vi "Rabi.vi"(6 "Gain":dbl=0.65, 7 "resolution (ns)":dbl=0.5, 9 "margin (ns)":i32=10, 11 "Pi pulse duration":dbl[unit]=5.000000000000001e-07) -> (2 "Array size":dbl=1280.0, 3 "Array":dbl[](array[numeric])=[0.0, 0.0, 0.0, 0.0, 0.0, 0.0, 0.0, 0.0, 0.0, 0.0, 0.0, 0.0, 0.0, 0.0, 0.0, 0.0, 0.0, 0.0, 0.0, 0.0, 0.325, 0.325, 0.325, 0.325, 0.325, 0.325, 0.325, 0.325, 0.325, 0.325, 0.325, 0.325, 0.325, 0.325, 0.325, 0.325, 0.325, 0.325, 0.325, 0.325, 0.325, 0.325, 0.325, 0.325, 0.325, 0.325, 0.325, 0.325, 0.325, 0.325, 0.325, 0.325, 0.325, 0.325, 0.325, 0.325, 0.325, 0.325, 0.325, 0.325, 0.325, 0.325, 0.325, 0.325, 0.325, 0.325, 0.325, 0.325, 0.325, 0.325, 0.325, 0.325, 0.325, 0.325, 0.325, 0.325, 0.325, 0.325, 0.325, 0.325, 0.325, 0.325, 0.325, 0.325, 0.325, 0.325, 0.325, 0.325, 0.325, 0.325, 0.325, 0.325, 0.325, 0.325, 0.325, 0.325, 0.325, 0.325, 0.325, 0.325, 0.325, 0.325, 0.325, 0.325, 0.325, 0.325, 0.325, 0.325, 0.325, 0.325, 0.325, 0.325, 0.325, 0.325, 0.325, 0.325, 0.325, 0.325, 0.325, 0.325, 0.325, 0.325, 0.325, 0.325, 0.325, 0.325, 0.325, 0.325, 0.325, 0.325, 0.325, 0.325, 0.325, 0.325, 0.325, 0.325, 0.325, 0.325, 0.325, 0.325, 0.325, 0.325, 0.325, 0.325, 0.325, 0.325, 0.325, 0.325, 0.325, 0.325, 0.325, 0.325, 0.325, 0.325, 0.325, 0.325, 0.325, 0.325, 0.325, 0.325, 0.325, 0.325, 0.325, 0.325, 0.325, 0.325, 0.325, 0.325, 0.325, 0.325, 0.325, 0.325, 0.325, 0.325, 0.325, 0.325, 0.325, 0.325, 0.325, 0.325, 0.325, 0.325, 0.325, 0.325, 0.325, 0.325, 0.325, 0.325, 0.325, 0.325, 0.325, 0.325, 0.325, 0.325, 0.325, 0.325, 0.325, 0.325, 0.325, 0.325, 0.325, 0.325, 0.325, 0.325, 0.325, 0.325, 0.325, 0.325, 0.325, 0.325, 0.325, 0.325, 0.325, 0.325, 0.325, 0.325, 0.325, 0.325, 0.325, 0.325, 0.325, 0.325, 0.325, 0.325, 0.325, 0.325, 0.325, 0.325, 0.325, 0.325, 0.325, 0.325, 0.325, 0.325, 0.325, 0.325, 0.325, 0.325, 0.325, 0.325, 0.325, 0.325, 0.325, 0.325, 0.325, 0.325, 0.325, 0.325, 0.325, 0.325, 0.325, 0.325, 0.325, 0.325, 0.325, 0.325, 0.325, 0.325, 0.325, 0.325, 0.325, 0.325, 0.325, 0.325, 0.325, 0.325, 0.325, 0.325, 0.325, 0.325, 0.325, 0.325, 0.325, 0.325, 0.325, 0.325, 0.325, 0.325, 0.325, 0.325, 0.325, 0.325, 0.325, 0.325, 0.325, 0.325, 0.325, 0.325, 0.325, 0.325, 0.325, 0.325, 0.325, 0.325, 0.325, 0.325, 0.325, 0.325, 0.325, 0.325, 0.325, 0.325, 0.325, 0.325, 0.325, 0.325, 0.325, 0.325, 0.325, 0.325, 0.325, 0.325, 0.325, 0.325, 0.325, 0.325, 0.325, 0.325, 0.325, 0.325, 0.325, 0.325, 0.325, 0.325, 0.325, 0.325, 0.325, 0.325, 0.325, 0.325, 0.325, 0.325, 0.325, 0.325, 0.325, 0.325, 0.325, 0.325, 0.325, 0.325, 0.325, 0.325, 0.325, 0.325, 0.325, 0.325, 0.325, 0.325, 0.325, 0.325, 0.325, 0.325, 0.325, 0.325, 0.325, 0.325, 0.325, 0.325, 0.325, 0.325, 0.325, 0.325, 0.325, 0.325, 0.325, 0.325, 0.325, 0.325, 0.325, 0.325, 0.325, 0.325, 0.325, 0.325, 0.325, 0.325, 0.325, 0.325, 0.325, 0.325, 0.325, 0.325, 0.325, 0.325, 0.325, 0.325, 0.325, 0.325, 0.325, 0.325, 0.325, 0.325, 0.325, 0.325, 0.325, 0.325, 0.325, 0.325, 0.325, 0.325, 0.325, 0.325, 0.325, 0.325, 0.325, 0.325, 0.325, 0.325, 0.325, 0.325, 0.325, 0.325, 0.325, 0.325, 0.325, 0.325, 0.325, 0.325, 0.325, 0.325, 0.325, 0.325, 0.325, 0.325, 0.325, 0.325, 0.325, 0.325, 0.325, 0.325, 0.325, 0.325, 0.325, 0.325, 0.325, 0.325, 0.325, 0.325, 0.325, 0.325, 0.325, 0.325, 0.325, 0.325, 0.325, 0.325, 0.325, 0.325, 0.325, 0.325, 0.325, 0.325, 0.325, 0.325, 0.325, 0.325, 0.325, 0.325, 0.325, 0.325, 0.325, 0.325, 0.325, 0.325, 0.325, 0.325, 0.325, 0.325, 0.325, 0.325, 0.325, 0.325, 0.325, 0.325, 0.325, 0.325, 0.325, 0.325, 0.325, 0.325, 0.325, 0.325, 0.325, 0.325, 0.325, 0.325, 0.325, 0.325, 0.325, 0.325, 0.325, 0.325, 0.325, 0.325, 0.325, 0.325, 0.325, 0.325, 0.325, 0.325, 0.325, 0.325, 0.325, 0.325, 0.325, 0.325, 0.325, 0.325, 0.325, 0.325, 0.325, 0.325, 0.325, 0.325, 0.325, 0.325, 0.325, 0.325, 0.325, 0.325, 0.325, 0.325, 0.325, 0.325, 0.325, 0.325, 0.325, 0.325, 0.325, 0.325, 0.325, 0.325, 0.325, 0.325, 0.325, 0.325, 0.325, 0.325, 0.325, 0.325, 0.325, 0.325, 0.325, 0.325, 0.325, 0.325, 0.325, 0.325, 0.325, 0.325, 0.325, 0.325, 0.325, 0.325, 0.325, 0.325, 0.325, 0.325, 0.325, 0.325, 0.325, 0.325, 0.325, 0.325, 0.325, 0.325, 0.325, 0.325, 0.325, 0.325, 0.325, 0.325, 0.325, 0.325, 0.325, 0.325, 0.325, 0.325, 0.325, 0.325, 0.325, 0.325, 0.325, 0.325, 0.325, 0.325, 0.325, 0.325, 0.325, 0.325, 0.325, 0.325, 0.325, 0.325, 0.325, 0.325, 0.325, 0.325, 0.325, 0.325, 0.325, 0.325, 0.325, 0.325, 0.325, 0.325, 0.325, 0.325, 0.325, 0.325, 0.325, 0.325, 0.325, 0.325, 0.325, 0.325, 0.325, 0.325, 0.325, 0.325, 0.325, 0.325, 0.325, 0.325, 0.325, 0.325, 0.325, 0.325, 0.325, 0.325, 0.325, 0.325, 0.325, 0.325, 0.325, 0.325, 0.325, 0.325, 0.325, 0.325, 0.325, 0.325, 0.325, 0.325, 0.325, 0.325, 0.325, 0.325, 0.325, 0.325, 0.325, 0.325, 0.325, 0.325, 0.325, 0.325, 0.325, 0.325, 0.325, 0.325, 0.325, 0.325, 0.325, 0.325, 0.325, 0.325, 0.325, 0.325, 0.325, 0.325, 0.325, 0.325, 0.325, 0.325, 0.325, 0.325, 0.325, 0.325, 0.325, 0.325, 0.325, 0.325, 0.325, 0.325, 0.325, 0.325, 0.325, 0.325, 0.325, 0.325, 0.325, 0.325, 0.325, 0.325, 0.325, 0.325, 0.325, 0.325, 0.325, 0.325, 0.325, 0.325, 0.325, 0.325, 0.325, 0.325, 0.325, 0.325, 0.325, 0.325, 0.325, 0.325, 0.325, 0.325, 0.325, 0.325, 0.325, 0.325, 0.325, 0.325, 0.325, 0.325, 0.325, 0.325, 0.325, 0.325, 0.325, 0.325, 0.325, 0.325, 0.325, 0.325, 0.325, 0.325, 0.325, 0.325, 0.325, 0.325, 0.325, 0.325, 0.325, 0.325, 0.325, 0.325, 0.325, 0.325, 0.325, 0.325, 0.325, 0.325, 0.325, 0.325, 0.325, 0.325, 0.325, 0.325, 0.325, 0.325, 0.325, 0.325, 0.325, 0.325, 0.325, 0.325, 0.325, 0.325, 0.325, 0.325, 0.325, 0.325, 0.325, 0.325, 0.325, 0.325, 0.325, 0.325, 0.325, 0.325, 0.325, 0.325, 0.325, 0.325, 0.325, 0.325, 0.325, 0.325, 0.325, 0.325, 0.325, 0.325, 0.325, 0.325, 0.325, 0.325, 0.325, 0.325, 0.325, 0.325, 0.325, 0.325, 0.325, 0.325, 0.325, 0.325, 0.325, 0.325, 0.325, 0.325, 0.325, 0.325, 0.325, 0.325, 0.325, 0.325, 0.325, 0.325, 0.325, 0.325, 0.325, 0.325, 0.325, 0.325, 0.325, 0.325, 0.325, 0.325, 0.325, 0.325, 0.325, 0.325, 0.325, 0.325, 0.325, 0.325, 0.325, 0.325, 0.325, 0.325, 0.325, 0.325, 0.325, 0.325, 0.325, 0.325, 0.325, 0.325, 0.325, 0.325, 0.325, 0.325, 0.325, 0.325, 0.325, 0.325, 0.325, 0.325, 0.325, 0.325, 0.325, 0.325, 0.325, 0.325, 0.325, 0.325, 0.325, 0.325, 0.325, 0.325, 0.325, 0.325, 0.325, 0.325, 0.325, 0.325, 0.325, 0.325, 0.325, 0.325, 0.325, 0.325, 0.325, 0.325, 0.325, 0.325, 0.325, 0.325, 0.325, 0.325, 0.325, 0.325, 0.325, 0.325, 0.325, 0.325, 0.325, 0.325, 0.325, 0.325, 0.325, 0.325, 0.325, 0.325, 0.325, 0.325, 0.325, 0.325, 0.325, 0.325, 0.325, 0.325, 0.325, 0.325, 0.325, 0.325, 0.325, 0.325, 0.325, 0.325, 0.325, 0.325, 0.325, 0.325, 0.325, 0.325, 0.325, 0.325, 0.325, 0.325, 0.325, 0.325, 0.325, 0.325, 0.325, 0.325, 0.325, 0.325, 0.325, 0.325, 0.325, 0.325, 0.325, 0.325, 0.325, 0.325, 0.325, 0.325, 0.325, 0.325, 0.325, 0.325, 0.325, 0.325, 0.325, 0.325, 0.325, 0.325, 0.325, 0.325, 0.325, 0.325, 0.325, 0.325, 0.325, 0.325, 0.325, 0.325, 0.325, 0.325, 0.325, 0.325, 0.325, 0.325, 0.325, 0.325, 0.325, 0.325, 0.325, 0.325, 0.325, 0.325, 0.325, 0.325, 0.325, 0.325, 0.325, 0.325, 0.325, 0.325, 0.325, 0.325, 0.325, 0.325, 0.325, 0.325, 0.325, 0.325, 0.325, 0.325, 0.325, 0.325, 0.325, 0.325, 0.325, 0.325, 0.325, 0.325, 0.325, 0.325, 0.325, 0.325, 0.325, 0.325, 0.325, 0.325, 0.325, 0.325, 0.325, 0.325, 0.325, 0.325, 0.0, 0.0, 0.0, 0.0, 0.0, 0.0, 0.0, 0.0, 0.0, 0.0, 0.0, 0.0, 0.0, 0.0, 0.0, 0.0, 0.0, 0.0, 0.0, 0.0, 0.0, 0.0, 0.0, 0.0, 0.0, 0.0, 0.0, 0.0, 0.0, 0.0, 0.0, 0.0, 0.0, 0.0, 0.0, 0.0, 0.0, 0.0, 0.0, 0.0, 0.0, 0.0, 0.0, 0.0, 0.0, 0.0, 0.0, 0.0, 0.0, 0.0, 0.0, 0.0, 0.0, 0.0, 0.0, 0.0, 0.0, 0.0, 0.0, 0.0, 0.0, 0.0, 0.0, 0.0, 0.0, 0.0, 0.0, 0.0, 0.0, 0.0, 0.0, 0.0, 0.0, 0.0, 0.0, 0.0, 0.0, 0.0, 0.0, 0.0, 0.0, 0.0, 0.0, 0.0, 0.0, 0.0, 0.0, 0.0, 0.0, 0.0, 0.0, 0.0, 0.0, 0.0, 0.0, 0.0, 0.0, 0.0, 0.0, 0.0, 0.0, 0.0, 0.0, 0.0, 0.0, 0.0, 0.0, 0.0, 0.0, 0.0, 0.0, 0.0, 0.0, 0.0, 0.0, 0.0, 0.0, 0.0, 0.0, 0.0, 0.0, 0.0, 0.0, 0.0, 0.0, 0.0, 0.0, 0.0, 0.0, 0.0, 0.0, 0.0, 0.0, 0.0, 0.0, 0.0, 0.0, 0.0, 0.0, 0.0, 0.0, 0.0, 0.0, 0.0, 0.0, 0.0, 0.0, 0.0, 0.0, 0.0, 0.0, 0.0, 0.0, 0.0, 0.0, 0.0, 0.0, 0.0, 0.0, 0.0, 0.0, 0.0, 0.0, 0.0, 0.0, 0.0, 0.0, 0.0, 0.0, 0.0, 0.0, 0.0, 0.0, 0.0, 0.0, 0.0, 0.0, 0.0, 0.0, 0.0, 0.0, 0.0, 0.0, 0.0, 0.0, 0.0, 0.0, 0.0, 0.0, 0.0, 0.0, 0.0, 0.0, 0.0, 0.0, 0.0, 0.0, 0.0, 0.0, 0.0, -0.325, -0.325, -0.325, -0.325, -0.325, -0.325, -0.325, -0.325, -0.325, -0.325, -0.325, -0.325, -0.325, -0.325, -0.325, -0.325, -0.325, -0.325, -0.325, -0.325, 0.0, 0.0, 0.0, 0.0, 0.0, 0.0, 0.0, 0.0, 0.0, 0.0, 0.0, 0.0, 0.0, 0.0, 0.0, 0.0, 0.0, 0.0, 0.0, 0.0, 0.0, 0.0, 0.0, 0.0, 0.0, 0.0, 0.0, 0.0, 0.0, 0.0, 0.0, 0.0, 0.0, 0.0, 0.0, 0.0, 0.0, 0.0, 0.0, 0.0])   [LabVIEW 2015]
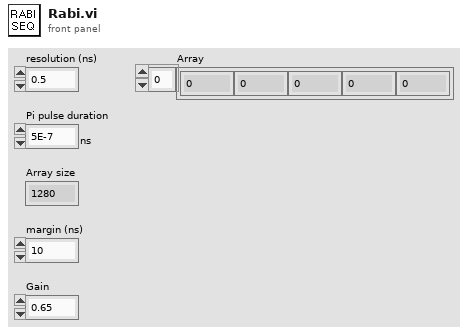
[diagram p1: front panel]
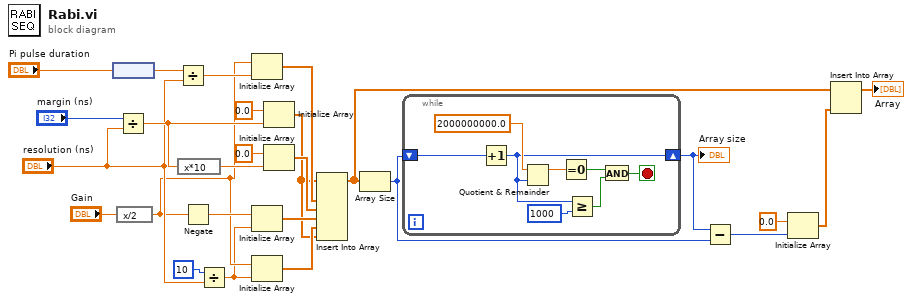
[diagram p0: block diagram]
diagram:
  n1 = node("Pi pulse duration") -> (w15:dbl)
  n2 = expression code="x/2"("Gain") -> (w4:dbl)
  n3 = Divide(x="margin (ns)", y="resolution (ns)") -> (x/y=w24:dbl)
  n4 = Divide(x=w15, y="resolution (ns)") -> (x/y=w23:dbl)
  n5 = expression code="x*10"(w24) -> (w18:dbl)
  n6 = Negate(x=w4) -> (-x=w21:dbl)
  n7 = Divide(x=10, y="resolution (ns)") -> (x/y=w3:dbl)
  n8 = Initialize Array(w4, w23) -> (w12:dbl[])
  n9 = Initialize Array(w21, w3) -> (w13:dbl[])
  n10 = Initialize Array(w4, w3) -> (w2:dbl[])
  n11 = Initialize Array(0.0 ("element"), w24) -> (w1:dbl[])
  n12 = Initialize Array(0.0 ("element"), w18) -> (w14:dbl[])
  n13 = Insert Into Array(array=w1, new element #1=w12, new element #2=w14, new element #3=w13, new element #4=w2, new element #5=w1) -> (w9:dbl[])  [unwired: 1 in]
  n14 = Array Size(array=w9) -> (size(s)=w16:i32)
  n15 = while {
    shift-right: [w28] -> w17
    shift-left: w16 -> [w34]
    stop <- w30 stop-if-true
    n16 = Increment(x=w34) -> (x+1=w28:i32)
    n17 = Quotient & Remainder(x=2000000000.0, y=w28) -> (x-y*floor(x/y)=w32:dbl)  [unwired: 1 out]
    n18 = Equal To 0?(x=w32) -> (x = 0?=w29:bool)
    n19 = Greater Or Equal?(x=w28, y=1000) -> (x >= y?=w31:bool)
    n20 = And(x=w29, y=w31) -> (x .and. y?=w30:bool)
  }
  "Array size" <- w17
  n21 = Subtract(x=w17, y=w16) -> (x-y=w11:i32)
  n22 = Initialize Array(0.0 ("element"), w11) -> (w8:dbl[])
  n23 = Insert Into Array(array=w9, new element=w8) -> (→"Array":dbl[])  [unwired: 1 in]
